vi "Path Notation Parse leading.vi"(11 "Item Path":string) -> (1 "End of Path":bool, 2 "<JSON>element names":string[](array[string]), 3 "Rest of Path":string)   [LabVIEW 2015, in "JSONtext.lvlib"]
uses:
  JSONtext.lvlib
  support/quote and escape json string 2.vi
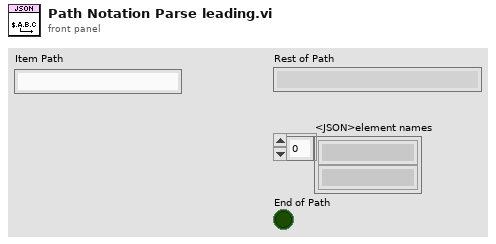
[diagram p1: front panel]
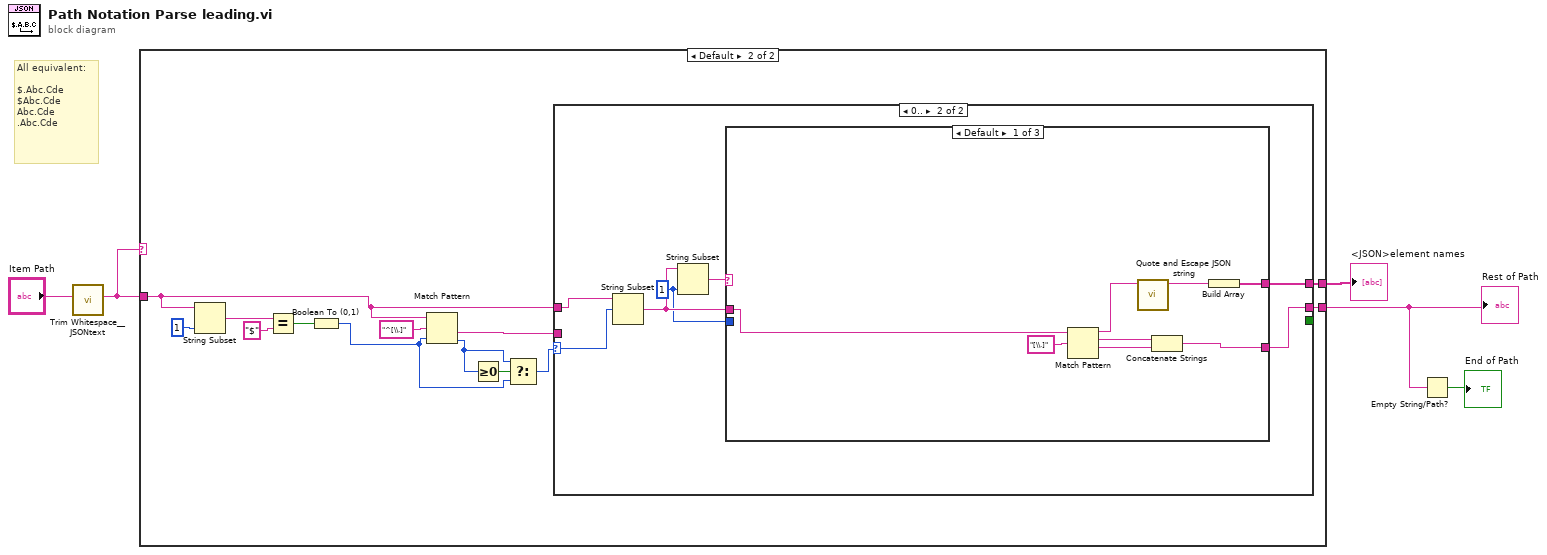
[diagram p0: block diagram]
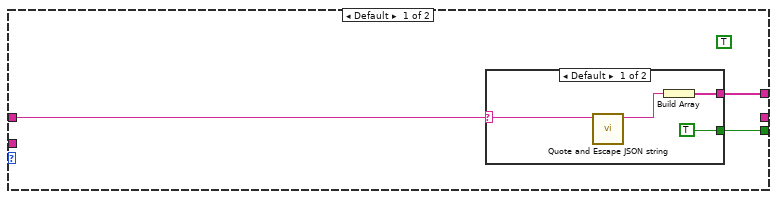
[diagram p3: hidden frame]
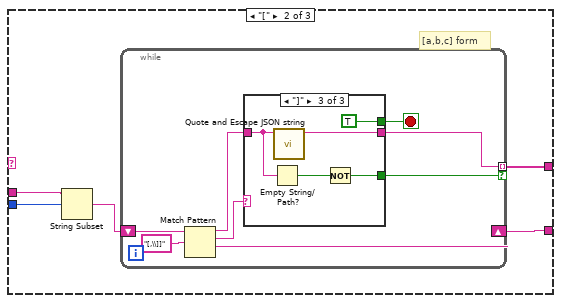
[diagram p5: hidden frame]
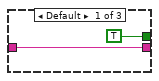
[diagram p6: hidden frame]
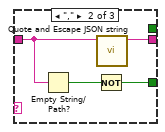
[diagram p7: hidden frame]
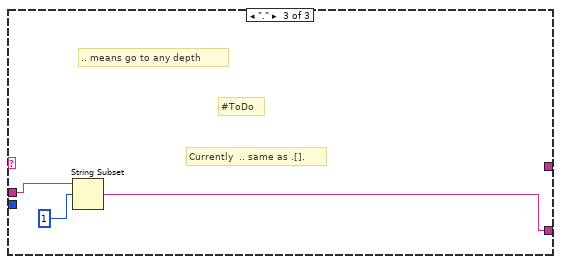
[diagram p8: hidden frame]
diagram:
  # "All equivalent:\n\n$.Abc.Cde\n$Abc.Cde\nAbc.Cde\n.Abc.Cde"
  n1 = call "Trim Whitespace__JSONtext.vi"("String in"="Item Path") -> ("String out"=w1:string)  [unwired: 6 in]
  n2 = case shown="Default" w1 {
    tunnel: [_ w12] -> w5
    tunnel: w1 -> [_ w7]
    tunnel: [_ w6] -> w3
    frame "" {
    }
    frame Default {
      n3 = String Subset(string=w7, length (rest)=1 ("length (rest)")) -> (substring=w18:string)  [unwired: 1 in]
      n4 = Equal?(x=w18, y="$") -> (x = y?=w15:bool)
      n5 = Boolean To (0,1)(Boolean=w15) -> (0, 1=w9:i16)
      n6 = Match Pattern(string=w7, regular expression="^[\\.]", offset (0)=w9) -> (after substring=w13:string, offset past match=w10:i32)  [unwired: 2 out]
      n7 = Greater Or Equal To 0?(x=w10) -> (x >= 0?=w11:bool)
      n8 = Select(t=w10, s=w11, f=w9) -> (s? t:f=w8:i32)
      n9 = case shown="0.." w8 {
        selector: w8 -> [_ w29]
        tunnel: [w20 w32] -> w12
        tunnel: [_ w31] -> w6
        tunnel: w13 -> [_ _]
        tunnel: [w19 _] -> _
        tunnel: w7 -> [w21 w30]
        frame Default {
          (unwired) TRUE
          n10 = case shown="Default" w21 {
            selector: w21 -> [w24 _]
            tunnel: [w23 _] -> w20
            tunnel: [TRUE _] -> w19
            frame Default {
              n11 = call "Quote and Escape JSON string.vi"("Plain Text"=w24) -> ("<JSON>"=w25:string)  [unwired: 10 in]
              n12 = Build Array(w25) -> (w23:string[])
            }
            frame "" {
            }
          }
        }
        frame 0.. {
          w26 = 1 ("length (rest)")
          n13 = String Subset(string=w30, offset (0)=w29) -> (substring=w27:string)  [unwired: 1 in]
          n14 = String Subset(string=w27, length (rest)=w26) -> (substring=w28:string)  [unwired: 1 in]
          n15 = case shown="Default" w28 {
            tunnel: [w37 w45 _] -> w32
            tunnel: [w35 w44 w66] -> w31
            tunnel: w27 -> [w33 w43 w65]
            tunnel: w26 -> [_ w42 _]
            frame Default {
              n16 = Match Pattern(string=w33, regular expression="[\\.]") -> (before substring=w39:string, match substring=w34:string, after substring=w36:string)  [unwired: 1 in, 1 out]
              n17 = call "Quote and Escape JSON string.vi"("Plain Text"=w39) -> ("<JSON>"=w38:string)  [unwired: 10 in]
              n18 = Concatenate Strings(w34, w36) -> (w35:string)
              n19 = Build Array(w38) -> (w37:string[])
            }
            frame "[" {
              # "[a,b,c] form"
              n20 = String Subset(string=w43, offset (0)=w42) -> (substring=w41:string)  [unwired: 1 in]
              n21 = while {
                tunnel: [w48] -> w45 mode=indexing if=w50
                shift-right: [w51] -> w44
                shift-left: w41 -> [w53]
                stop <- w46 stop-if-true
                n22 = Match Pattern(string=w53, regular expression="[,\\]]") -> (before substring=w49:string, match substring=w47:string, after substring=w51:string)  [unwired: 1 in, 1 out]
                n23 = case shown="\"]\"" w47 {
                  tunnel: [_ w58 w63] -> w50
                  tunnel: w49 -> [w54 w57 w62]
                  tunnel: [w54 w56 w61] -> w48
                  tunnel: [TRUE _ TRUE] -> w46
                  frame Default {
                  }
                  frame "," {
                    n24 = Empty String/Path?(string/path=w57) -> (empty?=w59:bool)
                    n25 = Not(x=w59) -> (.not. x?=w58:bool)
                    n26 = call "Quote and Escape JSON string.vi"("Plain Text"=w57) -> ("<JSON>"=w56:string)  [unwired: 10 in]
                  }
                  frame "]" {
                    n27 = Empty String/Path?(string/path=w62) -> (empty?=w64:bool)
                    n28 = call "Quote and Escape JSON string.vi"("Plain Text"=w62) -> ("<JSON>"=w61:string)  [unwired: 10 in]
                    n29 = Not(x=w64) -> (.not. x?=w63:bool)
                  }
                }
              }
            }
            frame "." {
              # "Currently  .. same as .[]."
              # "#ToDo"
              # ".. means go to any depth"
              n30 = String Subset(string=w65, offset (0)=1 ("length (rest)")) -> (substring=w66:string)  [unwired: 1 in]
            }
          }
        }
      }
    }
  }
  "Rest of Path" <- w3
  "<JSON>element names" <- w5
  n31 = Empty String/Path?(string/path=w3) -> (empty?=→"End of Path":bool)
